vi "RunOperation.vi"(10 "Inputs":string[](array[string]), 11 "Test in":refnum<class "Test.lvclass">) -> (1 "Output/Failure":string, 2 "CLI Process Return Code":i32, 3 "Test out":refnum<class "Test.lvclass">)   [LabVIEW 2017, in "Test.lvclass"]
uses:
  Test.lvclass
  LVUnit Test Discoverer/LVUnit Test Discoverer.lvclass
  LVUnit Test Executor/LVUnit Test Executor.lvclass
  C:/Users/pasca/Projects/Home/lvunit/Test Executor/Test Executor.lvclass
  Test.lvclass/Test.ctl
  Test Executor/Test Executor.lvclass
  CodeCoverage/CodeCoverage.lvclass
  Cobertura/Cobertura.lvlib
  JUnit/JUnit.lvlib
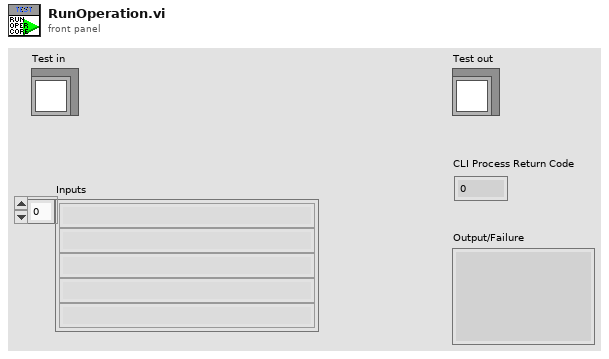
[diagram p1: front panel]
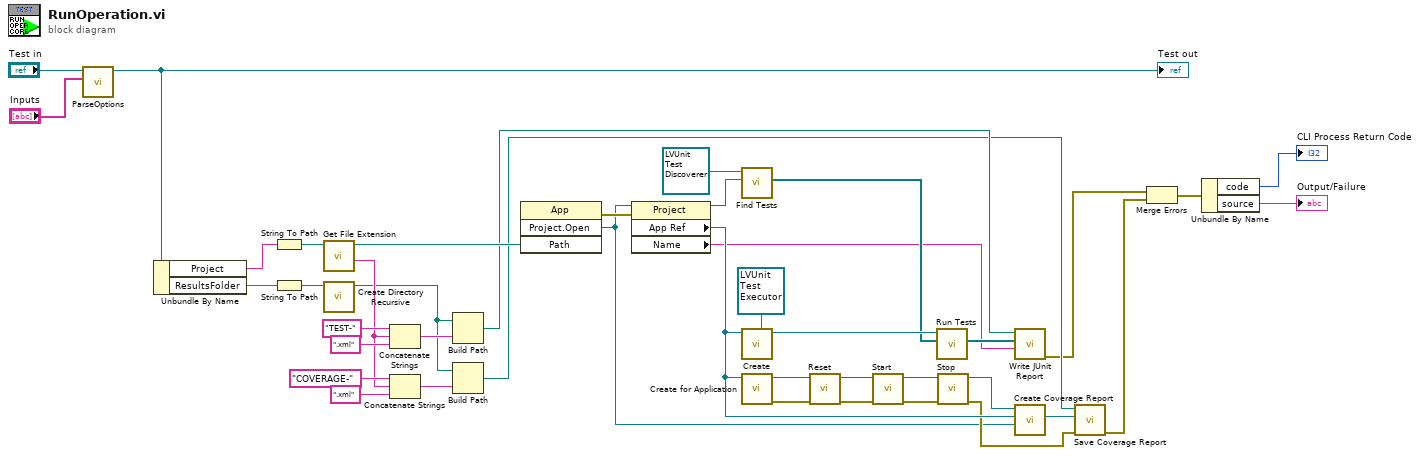
[diagram p0: block diagram]
diagram:
  n1 = call "ParseOptions.vi"("Options"="Inputs", "Test in"="Test in") -> ("Test out"=w38:refnum<class "Test.lvclass">)  [unwired: 8 in, 1 out]
  "Test out" <- w38
  n2 = Unbundle By Name(w38) -> ("Project"=w37:string, "ResultsFolder"=w35:string)
  n3 = String To Path(string=w37) -> (path=w33:path)
  n4 = String To Path(string=w35) -> (path=w34:path)
  n5 = call <vilib>:"Get File Extension.vi"("file"=w33) -> ("filename without extension"=w14:string, "dup file"=w29:path)  [unwired: 6 in, 3 out]
  n6 = call <vilib>:"Create Directory Recursive.vi"("directory"=w34) -> ("directory copy"=w12:path)  [unwired: 4 in, 2 out]
  n7 = Concatenate Strings("TEST-" ("string"), w14, ".xml" ("string")) -> (w30:string)
  n8 = Concatenate Strings("COVERAGE-" ("string"), w14, ".xml" ("string")) -> (w13:string)
  n9 = Build Path(base path=w12, name or relative path=w30) -> (appended path=w17:path)
  n10 = Build Path(base path=w12, name or relative path=w13) -> (appended path=w10:path)
  n11 = invoke class="App" method="Project.Open"("Path"=w29) -> (error out=w36:errorcluster, "Project:Open"=w1:refnum<vi>)  [unwired: 3 in, 2 out]
  n12 = property class="Project"(reference=w1, error in=w36) -> (reference out=w26:refnum<vi>, "App Ref"=w19:refnum<vi>, "Name"=w2:string)  [unwired: 1 out]
  n13 = call-dynamic "Find Tests.vi"("Project Refnum"=w26, "LVUnit Test Discoverer in"=refnum<class "LVUnit Test Discoverer.lvclass"> refnum ("LVUnit Test Discoverer")) -> ("Test Cases"=w22:refnum<class "Test Case.lvclass">[])  [unwired: 7 in, 2 out]
  n14 = call "Create.vi"("Test Executor in"=refnum<class "LVUnit Test Executor.lvclass"> refnum ("LVUnit Test Executor"), "Application"=w19) -> ("Test Executor"=w23:refnum<class "LVUnit Test Executor.lvclass">)  [unwired: 8 in, 1 out]
  n15 = call "Create for Application.vi"("Application"=w19) -> ("error out"=w3:errorcluster, "CodeCoverage out"=w24:refnum<class "CodeCoverage.lvclass">)  [unwired: 9 in]
  n16 = call "Reset.vi"("error in (no error)"=w3, "CodeCoverage in"=w24) -> ("error out"=w4:errorcluster, "CodeCoverage out"=w25:refnum<class "CodeCoverage.lvclass">)  [unwired: 8 in]
  n17 = call "Start.vi"("error in (no error)"=w4, "CodeCoverage in"=w25) -> ("error out"=w5:errorcluster, "CodeCoverage out"=w21:refnum<class "CodeCoverage.lvclass">)  [unwired: 8 in]
  n18 = call-dynamic "Run Tests.vi"("Test Cases"=w22, "LVUnit Test Executor in"=w23) -> ("Test Results"=w18:refnum<class "Test Result.lvclass">[])  [unwired: 7 in, 2 out]
  n19 = call "Stop.vi"("error in (no error)"=w5, "CodeCoverage in"=w21) -> ("error out"=w6:errorcluster, "CodeCoverage out"=w20:refnum<class "CodeCoverage.lvclass">)  [unwired: 8 in]
  n20 = call "Write JUnit Report.vi"("Project Name"=w2, "Test Results"=w18, "File Path"=w17) -> ("error out"=w8:errorcluster)  [unwired: 8 in]
  n21 = call "Create Coverage Report.vi"("Project"=w1, "Application"=w19, "CodeCoverage in"=w20) -> ("Coverage"=w11:refnum<class "Coverage.lvclass">)  [unwired: 7 in, 1 out]
  n22 = call "Save Coverage Report.vi"("error in (no error)"=w6, "Coverage"=w11, "Path"=w10) -> ("error out"=w7:errorcluster)  [unwired: 8 in]
  n23 = Merge Errors(w8, w7) -> (w9:errorcluster)
  n24 = Unbundle By Name(w9) -> ("code"=→"CLI Process Return Code":i32, "source"=→"Output/Failure":string)
